vi "dfd_X Eaual Zero.vi"(0 "x":dbl=1.0, 1 "tolerance":dbl=1e-12) -> (2 "equal?":bool)   [LabVIEW 2017, in "NI_DigFilterLicensed.lvlib"]
uses:
  <vilib>/addons/Digital Filter Design/NI_DigFilterLicensed.lvlib
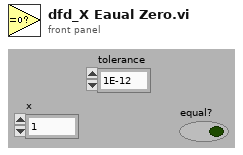
[diagram p1: front panel]
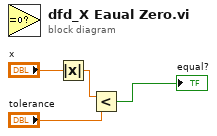
[diagram p0: block diagram]
diagram:
  n1 = Absolute Value(x="x") -> (abs(x)=w2:dbl)
  n2 = Less?(x=w2, y="tolerance") -> (x < y?=→"equal?":bool)
